vi "Untitled 2 (SubVI).vi"(0 "Количество \nЭлеметнов":dbl, 1 "Множитель":dbl, 3 "Первый\nчлен":dbl) -> (2 "Array":dbl[](array[numeric]), 4 "Сумма":dbl)   [LabVIEW 2021]
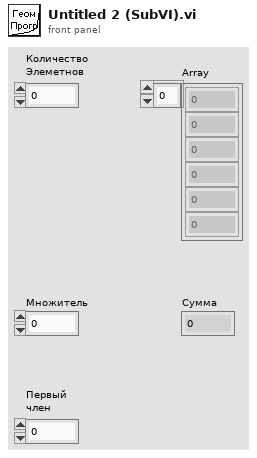
[diagram p1: front panel]
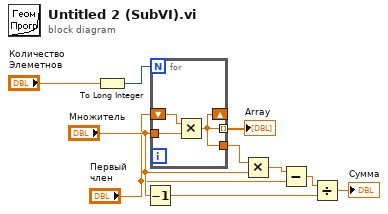
[diagram p0: block diagram]
diagram:
  n1 = To Long Integer(number="Количество \nЭлеметнов") -> (32bit integer=w2:i32)
  n2 = Decrement(x="Множитель") -> (x-1=w9:dbl)
  n3 = for {
    N: w2 -> [_]
    shift-right: [w11] -> _
    shift-left: "Первый\nчлен" -> [w13]
    tunnel: "Множитель" -> [w12]
    tunnel: [w11] -> w1 mode=indexing
    tunnel: [w11] -> w4
    n4 = Multiply(x=w13, y=w12) -> (x*y=w11:dbl)
  }
  "Array" <- w1
  n5 = Multiply(x=w4, y="Множитель") -> (x*y=w5:dbl)
  n6 = Subtract(x=w5, y="Первый\nчлен") -> (x-y=w7:dbl)
  n7 = Divide(x=w7, y=w9) -> (x/y=→"Сумма":dbl)
